vi "DataVIS_Parse Sweep Control JSON.vi"(8 "error in (no error)":errorcluster, 11 "File Information":T9={"File or folder path (input)"=path "G:/My Drive/ansom/Data/Agilent/TEST.20190618/6H_IVcurves", "output file description"="fakedata_test"}) -> (0 "error out":errorcluster, 1 "sweep dimensions":i32, 2 "json path":path, 3 "Sorted Sweep Info":T8 {"Sorted scan parameters"."?"."Rate" format="%.2f"; "Sorted scan parameters"."?"."Step" format="%#_6p"; "Sorted scan parameters"."?"."End" format="%#_6p"; "Sorted scan parameters"."?"."Start" format="%#_6p"}, 4 "sweep scan names":T1[](array[typedef]), 5 "sweep sizes":i32[](array[numeric]), 6 "sweep scan names (strings)":string[](array[string]))   [LabVIEW 2016]
uses:
  <userlib>/LevyLab/Transport/SweepControl/Typedefs/ScanControl.ctl
  <userlib>/LevyLab/Transport/SweepControl/Typedefs/Cluster - ScanControl.ctl
  <userlib>/LevyLab/Transport/SweepControl/Typedefs/Enum - Priority.ctl
  <userlib>/LevyLab/Transport/SweepControl/Typedefs/Enum - Action.ctl
  <userlib>/LevyLab/Transport/SweepControl/Typedefs/ScanParamters.ctl
  <userlib>/LevyLab/Transport/SweepControl/Typedefs/Cluster - ScanParamters.ctl
  <userlib>/LevyLab/Transport/SweepControl/Typedefs/Enum - Experiments.ctl
  <userlib>/LevyLab/Transport/SweepControl/Typedefs/Sweep Control Configuration--Cluster.ctl
  <userlib>/LevyLab/Transport/SweepControl/SweepControl.lvclass
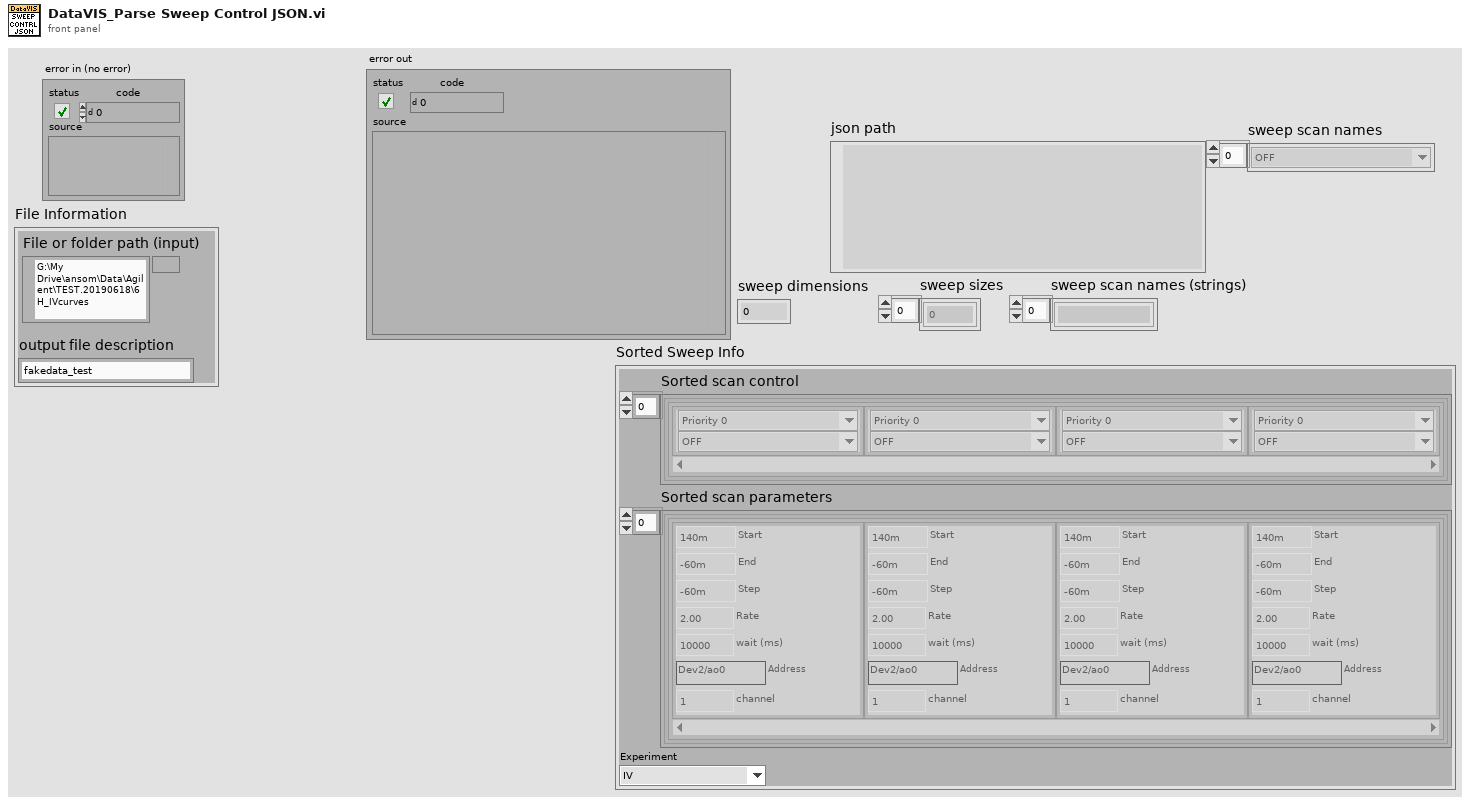
[diagram p1: front panel]
types:
  T1 = typedef "SweepControl.lvclass/Enum - Action.ctl" = enum16{"OFF", "DSA_Vamp", "DSA_freq", "DSA_Vsg1", "DSA_Vsg2", "DSA_Vsg3", "DAQ_Vbg", "B_Field", "Humidity", "Temp", "MW_freq1", "MW_freq2", "MW_amplitude1", "MW_amplitude2"}
  T2 = typedef "SweepControl.lvclass/ScanControl.ctl" = T3[]
  T3 = typedef "SweepControl.lvclass/Cluster - ScanControl.ctl" = cluster{"Priority":T4, "Scan name":T1}
  T4 = typedef "SweepControl.lvclass/Enum - Priority.ctl" = enum16{"Priority 0", "Priority 1", "Priority 2", "Priority 3", "Priority 4", "Priority 5"}
  T5 = typedef "SweepControl.lvclass/ScanParamters.ctl" = T6[]
  T6 = typedef "SweepControl.lvclass/Cluster - ScanParamters.ctl" = cluster{"Start":dbl, "End":dbl, "Step":dbl, "Rate":dbl, "wait (ms)":u32, "Address":string, "channel":i32}
  T7 = typedef "SweepControl.lvclass/Enum - Experiments.ctl" = enum16{"IV", "Lockin_time", "Lockin_Vsg", "Lockin (experimental)", "Lockin_Vsg_JKISM"}
  T8 = cluster{"Sorted scan control":cluster{T2}[], "Sorted scan parameters":cluster{T5}[], "Experiment":T7}
  T9 = cluster{"File or folder path (input)":path, "output file description":string}
  T10 = typedef "SweepControl.lvclass/Sweep Control Configuration--Cluster.ctl" = cluster{"Scan control":T2, "Scan parameters":T5, "Experiment":T7}
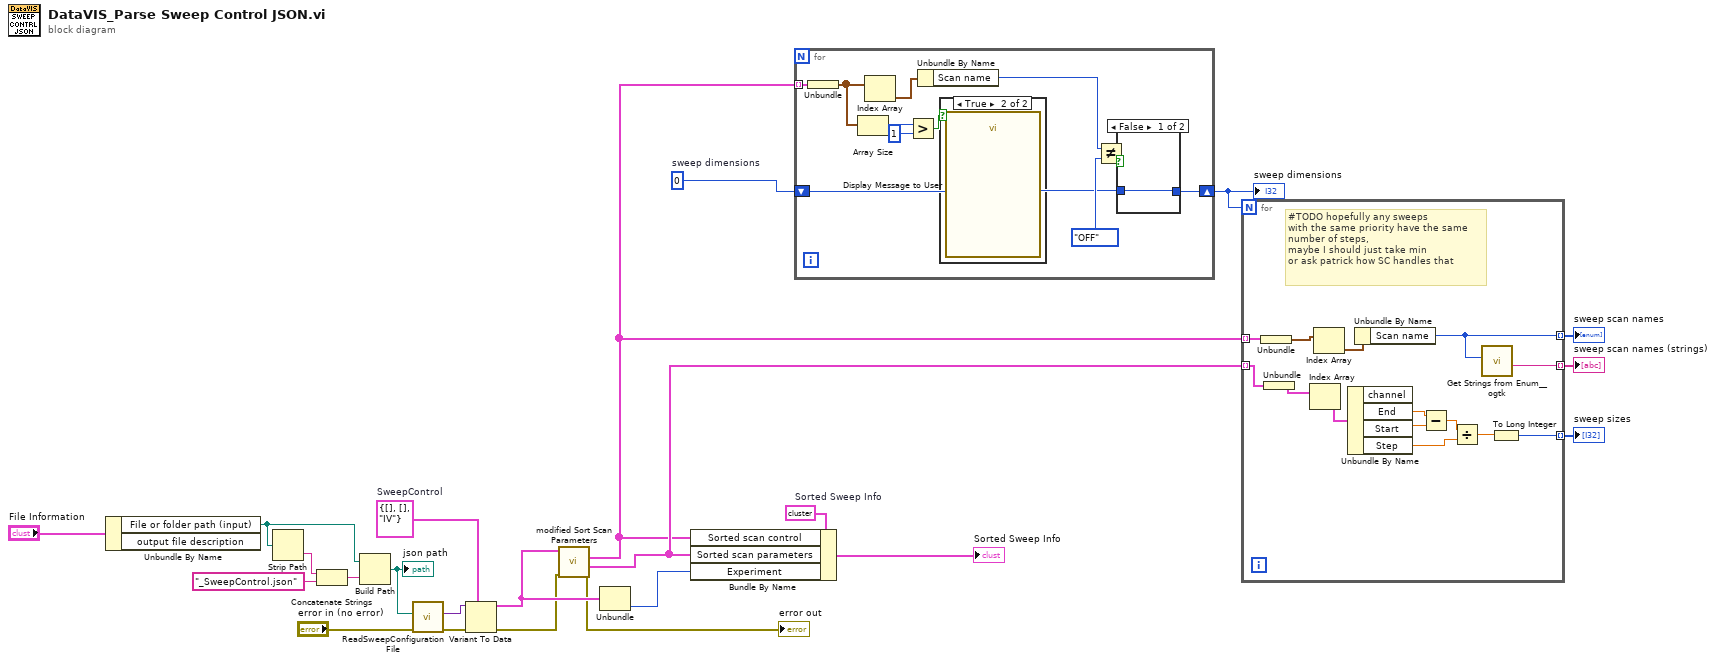
[diagram p0: block diagram]
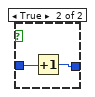
[diagram p2: hidden frame]
diagram:
  w7 = 0  # sweep dimensions
  w10 = T8 {"Sorted scan control"=[{[{"Priority"=enum."Priority 0", "Scan name"=enum."DSA_Vsg2"}]}, {[{"Priority"=enum."Priority 1", "Scan name"=enum."DSA_Vamp"}]}, {[{"Priority"=enum."Priority 2", "Scan name"=enum."DSA_Vsg1"}, {"Priority"=enum."Priority 2", "Scan name"=enum."DSA_Vsg3"}]}], "Sorted scan parameters"=[{[{"Start"=0.14, "End"=-0.060000000000000005, "Step"=-0.060000000000000005, "Rate"=0.0, "wait (ms)"=10000, "Address"="Dev2/ao0", "channel"=1}]}, {[{"Start"=0.14, "End"=-0.060000000000000005, "Step"=-0.060000000000000005, "Rate"=0.0, "wait (ms)"=10000, "Address"="Dev2/ao0", "channel"=1}]}, {[{"Start"=0.14, "End"=-0.060000000000000005, "Step"=-0.060000000000000005, "Rate"=0.0, "wait (ms)"=10000, "Address"="Dev2/ao0", "channel"=1}, {"Start"=0.14, "End"=-0.060000000000000005, "Step"=-0.060000000000000005, "Rate"=0.0, "wait (ms)"=10000, "Address"="Dev2/ao0", "channel"=1}]}], "Experiment"=enum."Lockin_Vsg"}  # Sorted Sweep Info
  w21 = T10 {"Scan control"=[], "Scan parameters"=[], "Experiment"=enum."IV"}  # SweepControl
  n1 = Unbundle By Name("File Information") -> ("File or folder path (input)"=w17:path)  [unwired: 1 out]
  n2 = Strip Path(path=w17) -> (name=w19:string)  [unwired: 1 out]
  n3 = Concatenate Strings(w19, "_SweepControl.json") -> (w16:string)
  n4 = Build Path(base path=w17, name or relative path=w16) -> (appended path=w15:path)
  "json path" <- w15
  n5 = call <userlib>:"ReadSweepConfigurationFile.vi"("error in (no error)"="error in (no error)", "Path"=w15) -> ("error out"=w23:errorcluster, "Data"=w22:variant)  [unwired: 7 in, 1 out]
  n6 = Variant To Data(error in=w23, type=w21, Variant=w22) -> (data=w13:T10, error out=w12:errorcluster)
  n7 = call "modified Sort Scan Parameters.vi"("error in (no error)"=w12, "data"=w13) -> ("error out"=→"error out":errorcluster, "Sorted scan parameters"=w5:cluster{T5}[], "Sorted scan control"=w3:cluster{T2}[])  [unwired: 7 in]
  n8 = Unbundle(w13) -> ("Experiment"=w9:T7)  [unwired: 2 out]
  n9 = Bundle By Name(cluster=w10, "Sorted scan control"=w3, "Sorted scan parameters"=w5, "Experiment"=w9) -> (→"Sorted Sweep Info":T8)
  n10 = for {
    tunnel: w3 -> [w34] mode=indexing
    shift-right: [w25] -> w6
    shift-left: w7 -> [w26]
    n11 = Unbundle(w34) -> (w33:T2)
    n12 = Array Size(array=w33) -> (size(s)=w32:i32)
    n13 = Index Array(array=w33) -> (element=w29:T3)  [unwired: 1 in]
    n14 = Greater?(x=w32, y=1) -> (0:w30:bool)
    n15 = Unbundle By Name(w29) -> ("Scan name"=w27:T1)
    n16 = case shown="True" w30 {
      frame False {
      }
      frame True {
        n17 = call "Display Message to User"() -> ()  [unwired: 10 in, 2 out]
      }
    }
    n18 = Not Equal?(x=w27, y=Enum_-_Action."OFF" ("Scan name")) -> (x != y?=w24:bool)
    n19 = case shown="False" w24 {
      tunnel: w26 -> [w35 w37]
      tunnel: [w35 w36] -> w25
      frame False {
      }
      frame True {
        n20 = Increment(x=w37) -> (x+1=w36:i32)
      }
    }
  }
  "sweep dimensions" <- w6
  n21 = for {
    N: w6 -> [_]
    tunnel: w5 -> [w51] mode=indexing
    tunnel: [w43] -> w4 mode=indexing
    tunnel: w3 -> [w42] mode=indexing
    tunnel: [w39] -> w2 mode=indexing
    tunnel: [w38] -> w1 mode=indexing
    # "#TODO hopefully any sweeps\nwith the same priority have the same \nnumber of steps,\nmaybe I should just take min\nor ask patrick how SC handles that"
    n22 = Unbundle(w42) -> (w41:T2)
    n23 = Unbundle(w51) -> (w50:T5)
    n24 = Index Array(array=w50) -> (element=w49:T6)  [unwired: 1 in]
    n25 = Index Array(array=w41) -> (element=w40:T3)  [unwired: 1 in]
    n26 = Unbundle By Name(w49) -> ("End"=w48:dbl, "Start"=w47:dbl, "Step"=w45:dbl)  [unwired: 1 out]
    n27 = Unbundle By Name(w40) -> ("Scan name"=w39:T1)
    n28 = Subtract(x=w48, y=w47) -> (x-y=w46:dbl)
    n29 = Divide(x=w46, y=w45) -> (x/y=w44:dbl)
    n30 = call <userlib>:"Get Strings from Enum__ogtk.vi"("Enum"=w39) -> ("String Value"=w38:string)  [unwired: 7 in, 3 out]
    n31 = To Long Integer(number=w44) -> (32bit integer=w43:i32)
  }
  "sweep sizes" <- w4
  "sweep scan names" <- w2
  "sweep scan names (strings)" <- w1
